vi "Initialize.vi"(8 "error in":errorcluster, 10 "shared resources":refnum<class "Shared Resources.lvclass">, 11 "AIM ARINC-429 logging execution unit in":refnum<class "Logging Execution Unit.lvclass">) -> (0 "error out":errorcluster, 3 "AIM ARINC-429 logging execution unit out":refnum<class "Logging Execution Unit.lvclass">)   [LabVIEW 2020, in "AIM ARINC 429 Engine.lvlib" / "Implementation.lvlib" / "Logging Execution Unit.lvclass"]
uses:
  Logging Execution Unit.lvclass
  C:/Git/niveristand-aim-arinc429-custom-device/Source/Custom Device Support/Engine/Implementation/Execution Unit/Execution Unit.lvclass
  Interfaces/Shared Resources/Shared Resources.lvclass
  Shared Resources/Shared Resources.lvclass
  <instrlib>/AIM GmbH/ARINC-429/Session/controls/api429_rm_setup.ctl
  <instrlib>/AIM GmbH/ARINC-429/Session/controls/rm_setup_mode.ctl
  <instrlib>/AIM GmbH/ARINC-429/Session/controls/rm_setup_interrupt_mode.ctl
  Shared Resources/Shared Resources.lvclass/Shared Resources.ctl
  Execution Unit/Execution Unit.lvclass/Execution Unit.ctl
  Logging Execution Unit.lvclass/Logging Execution Unit.ctl
  <instrlib>/AIM GmbH/ARINC-429/subvi/Error Converter (ErrCode or Status).vi
  <instrlib>/AIM GmbH/ARINC-429/subvi/Get Library Path.vi
  <instrlib>/AIM GmbH/ARINC-429/VIs/Library/Api429Lib Error Desc Get.vi
  <instrlib>/AIM GmbH/ARINC-429/subvi/Get Error Number Offset.vi
  <vilib>/Utility/error.llb/Error Cluster From Error Code.vi
  <instrlib>/AIM GmbH/ARINC-429/AIM429LV.lvlib
  Execution Unit/Execution Unit.lvclass
  <instrlib>/AIM GmbH/ARINC-429/Session/Session.lvclass
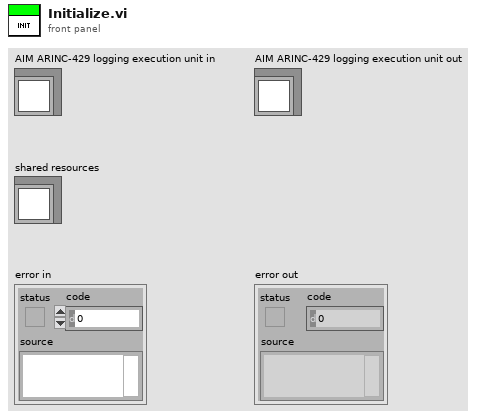
[diagram p1: front panel]
types:
  T1 = cluster{"mode":i32, "size_in_entries":u32, "tat_count":u32, "interrupt_mode":i32}
  T2 = typedef "AIM429LV.lvlib/Session.lvclass/api429_rm_setup.ctl" = cluster{"mode":T3, "size in entries":u32, "trace after trigger count":u32, "interrupt mode":T4}
  T3 = typedef "AIM429LV.lvlib/Session.lvclass/rm_setup_mode.ctl" = i8
  T4 = typedef "AIM429LV.lvlib/Session.lvclass/rm_setup_interrupt_mode.ctl" = i8
  T5 = typedef "AIM ARINC 429 Engine.lvlib/Custom Device.lvlib/Hardware Handles.ctl" = cluster{"module":u8}
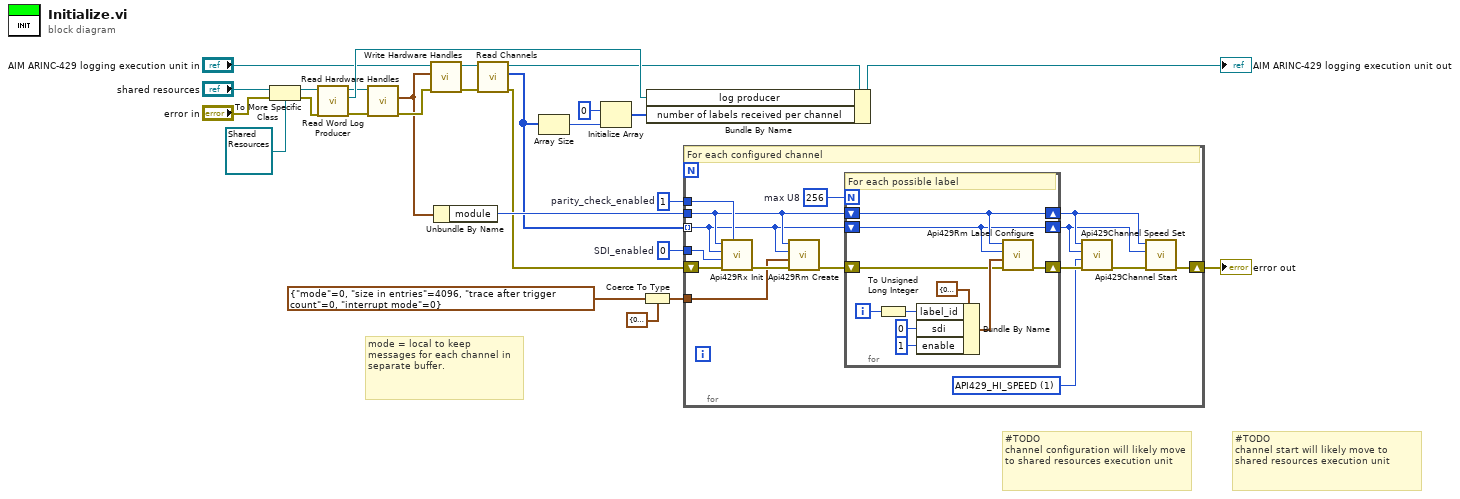
[diagram p0: block diagram]
diagram:
  w18 = u8 1  # parity_check_enabled
  w19 = u8 0  # SDI_enabled
  # "#TODO\nchannel start will likely move to shared resources execution unit"
  # "#TODO\nchannel configuration will likely move to shared resources execution unit"
  # "mode = local to keep messages for each channel in separate buffer."
  n1 = To More Specific Class(target class=refnum<class "Shared Resources.lvclass"> refnum ("AIM ARINC-429 shared resources in"), reference="shared resources", error in="error in") -> (specific class reference=w5:refnum<class "Shared Resources.lvclass">, error out=w4:errorcluster)
  n2 = call-dynamic "Read Word Log Producer.vi"("error in"=w4, "shared resources in"=w5) -> ("error out"=w3:errorcluster, "word log producer"=w23:refnum<class "Log Producer.lvclass">, "shared resources out"=w1:refnum<class "Shared Resources.lvclass">)  [unwired: 7 in]
  n3 = call "Read Hardware Handles.vi"("error in"=w3, "AIM ARINC-429 shared resources in"=w1) -> ("error out"=w24:errorcluster, "hardware handles"=w21:T5)  [unwired: 7 in, 1 out]
  n4 = call "Write Hardware Handles.vi"("error in"=w24, "hardware handles"=w21, "AIM ARINC-429 execution unit in"="AIM ARINC-429 logging execution unit in") -> ("error out"=w10:errorcluster, "AIM ARINC-429 execution unit out"=w12:refnum<class "Logging Execution Unit.lvclass">)  [unwired: 7 in]
  n5 = Unbundle By Name(w21) -> ("module"=w20:u8)
  n6 = call "Read Channels.vi"("error in"=w10, "execution unit in"=w12) -> ("error out"=w2:errorcluster, "channels"=w9:u8[], "execution unit out"=w11:refnum<class "Logging Execution Unit.lvclass">)  [unwired: 7 in]
  n7 = Array Size(array=w9) -> (size(s)=w8:i32)
  n8 = Initialize Array(u64 0 ("element"), w8) -> (w6:u64[])
  n9 = Coerce To Type(0:T2 {"mode"=0, "size in entries"=4096, "trace after trigger count"=0, "interrupt mode"=0} ("receive monitor setup"), 1:T1 {"mode"=0, "size_in_entries"=0, "tat_count"=0, "interrupt_mode"=0} ("setup")) -> (2:w15:T1)
  n10 = Bundle By Name(cluster=w11, "log producer"=w23, "number of labels received per channel"=w6) -> (→"AIM ARINC-429 logging execution unit out":refnum<class "Logging Execution Unit.lvclass">)
  n11 = for {
    tunnel: w9 -> [w36] mode=indexing
    tunnel: w20 -> [w37]
    tunnel: w19 -> [w42]
    tunnel: w18 -> [w39]
    tunnel: w15 -> [w38]
    shift-right: [w30] -> w14
    shift-left: w2 -> [w41]
    w32 = u32 1 items=["API429_LO_SPEED", "API429_HI_SPEED"] ("speed")
    w35 = 256  # max U8
    # "For each configured channel"
    n12 = call <instrlib>:"Api429Rx Init.vi"("parity_check_enabled"=w39, "error in (no error)"=w41, "sdi_enabled"=w42, "b_Chn"=w36, "board_handle"=w37) -> ("error out"=w40:errorcluster)  [unwired: 6 in]
    n13 = call <instrlib>:"Api429Rm Create.vi"("error in (no error)"=w40, "setup"=w38, "channel_id"=w36, "board_handle"=w37) -> ("error out"=w34:errorcluster)  [unwired: 7 in]
    n14 = for {
      N: w35 -> [_]
      shift-right: [w45] -> w33
      shift-left: w34 -> [w46]
      shift-right: [w44] -> w29
      shift-left: w37 -> [w44]
      shift-right: [w43] -> w28
      shift-left: w36 -> [w43]
      i -> [w51]
      # "For each possible label"
      n15 = To Unsigned Long Integer(number=w51) -> (unsigned 32bit integer=w50:u32)
      n16 = Bundle By Name(cluster=cluster{"label_id":u32, "sdi":u32, "enable":u8} {"label_id"=0, "sdi"=0, "enable"=1} ("label_config"), "label_id"=w50, "sdi"=u32 0, "enable"=u8 1) -> (w47:cluster{"label_id":u32, "sdi":u32, "enable":u8})
      n17 = call <instrlib>:"Api429Rm Label Configure.vi"("error in (no error)"=w46, "label_config"=w47, "b_Chn"=w43, "board_handle"=w44) -> ("error out"=w45:errorcluster)  [unwired: 7 in]
    }
    n18 = call <instrlib>:"Api429Channel Speed Set.vi"("error in (no error)"=w33, "speed"=w32, "b_Chn"=w28, "board_handle"=w29) -> ("error out"=w31:errorcluster)  [unwired: 7 in]
    n19 = call <instrlib>:"Api429Channel Start.vi"("error in (no error)"=w31, "channel_id"=w28, "board_handle"=w29) -> ("error out"=w30:errorcluster)  [unwired: 8 in]
  }
  "error out" <- w14
